vi "Read Datatype Children Information.vi"(8 "error in (no error)":errorcluster, 10 "Parent Name":string, 11 "TwinCAT ADS in":refnum<class "TwinCAT ADS.lvclass">) -> (0 "error out":errorcluster, 1 "Datatype Children Information":T1[](array[typedef]) {"Category" items=["Unknown, None"=0, "Primitive"=1, "Alias"=2, "Enum"=3, "Array"=4, "Struct"=5, "FunctionBlock"=6, "Program"=7, "Function"=8, "SubRange"=9, "String"=10, "Bitset"=12, "Pointer"=13, "Union"=14, "Reference"=15, "Interface"=16]; "Type ID" items=["ADST_VOID"=0, "ADST_INT16"=2, "ADST_INT32"=3, "ADST_REAL32"=4, "ADST_REAL64"=5, "ADST_INT8"=16, "ADST_UINT8"=17, "ADST_UINT16"=18, "ADST_UINT32"=19, "ADST_INT64"=20, "ADST_UINT64"=21, "ADST_STRING"=30, "ADST_WSTRING"=31, "ADST_REAL80"=32, "ADST_BIT"=33, "ADST_MAXTYPES"=34, "ADST_BIGTYPE"=65]}, 3 "TwinCAT ADS out":refnum<class "TwinCAT ADS.lvclass">)   [LabVIEW 2018, in "TwinCAT ADS.lvclass"]
uses:
  TwinCAT ADS.lvclass
  Controls/Datatype Child Information.ctl
  TwinCAT.Ads
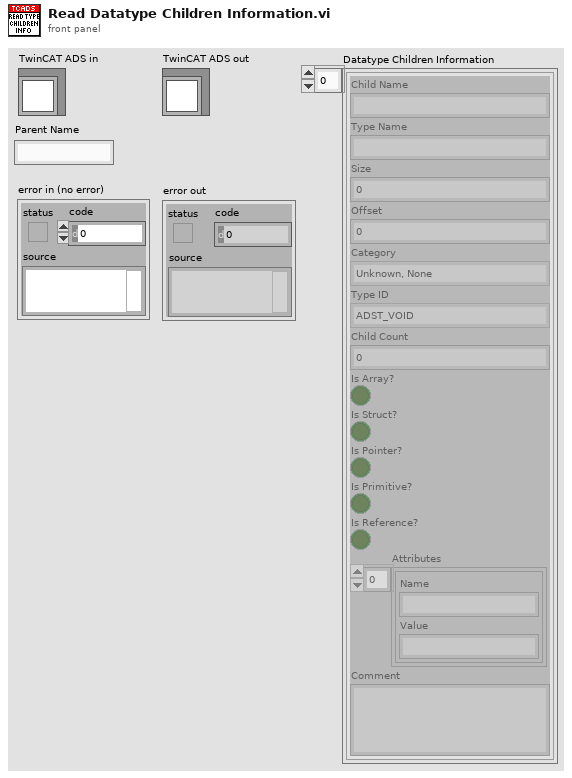
[diagram p1: front panel]
types:
  T1 = typedef "TwinCAT ADS.lvclass/Datatype Child Information.ctl" = cluster{"Child Name":string, "Type Name":string, "Size":i32, "Offset":i32, "Category":i32, "Type ID":i32, "Child Count":i32, "Is Array?":bool, "Is Struct?":bool, "Is Pointer?":bool, "Is Primitive?":bool, "Is Reference?":bool, "Attributes":cluster{"Name":string, "Value":string}[], "Comment":string}
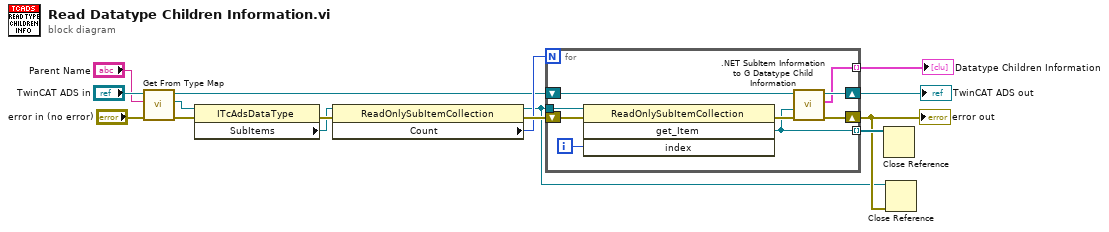
[diagram p0: block diagram]
diagram:
  n1 = call "Get From Type Map.vi"("error in (no error)"="error in (no error)", "Type Name"="Parent Name", "TwinCAT ADS in"="TwinCAT ADS in") -> ("error out"=w12:errorcluster, ".NET AdsDataType"=w11:refnum<k24>, "TwinCAT ADS out"=w6:refnum<class "TwinCAT ADS.lvclass">)  [unwired: 6 in]
  n2 = property class="ITcAdsDataType"(reference=w11, error in=w12) -> (error out=w10:errorcluster, "SubItems"=w9:refnum<k24>)  [unwired: 1 out]
  n3 = property class="ReadOnlySubItemCollection"(reference=w9, error in=w10) -> (reference out=w2:refnum<k24>, error out=w8:errorcluster, "Count"=w7:i32)
  n4 = for {
    N: w7 -> [_]
    shift-right: [w18] -> w5
    shift-left: w6 -> [w20]
    shift-right: [w17] -> w3
    shift-left: w8 -> [w24]
    tunnel: w2 -> [w23]
    tunnel: [w19] -> w4 mode=indexing
    tunnel: [w16] -> w1 mode=indexing
    i -> [w22]
    n5 = invoke class="ReadOnlySubItemCollection" method="get_Item"(reference=w23, error in=w24, "index"=w22) -> (error out=w21:errorcluster, "get_Item"=w19:refnum<k24>)  [unwired: 1 in, 2 out]
    n6 = call ".NET SubItem Information to G Datatype Child Information.vi"("error in (no error)"=w21, ".NET AdsSubItem"=w19, "TwinCAT ADS in"=w20) -> ("error out"=w17:errorcluster, "Datatype Child Information"=w16:T1, "TwinCAT ADS out"=w18:refnum<class "TwinCAT ADS.lvclass">)  [unwired: 6 in]
  }
  "error out" <- w3
  "TwinCAT ADS out" <- w5
  "Datatype Children Information" <- w1
  n7 = Close Reference(reference=w4) -> ()  [unwired: 1 in, 1 out]
  n8 = Close Reference(reference=w2, error in (no error)=w3) -> ()  [unwired: 1 out]
